vi "Actor Core.vi"(8 "error in":errorcluster, 11 "[V] User List in":refnum<class "[V] User List.lvclass">) -> (0 "error out":errorcluster, 3 "Actor out":refnum<class "Actor.lvclass">)   [LabVIEW 2020, in "[V] User List.lvlib" / "[V] User List.lvclass"]
doc: "(<B>Filename</B>: Actor Framework.lvlib:Actor.lvclass:Actor Core.vi)\n\nReceives messages to the actor, reacts to them, and initiates any error handling that may shut the actor down.\n\nDescendant classes may override this VI to append parallel tasks for the actor to complete while it handles messages. Overrides use the Call Parent Class Method node."
uses:
  [V] User List.lvclass
  C:/Program Files (x86)/National Instruments/LabVIEW 2020/vi.lib/ActorFramework/Actor/Actor.lvclass
  <vilib>/ActorFramework/Actor/Actor.lvclass
  Control/New User.ctl
  Control/Delete User.ctl
  <vilib>/ActorFramework/Actor/Actor.lvclass/Actor.ctl
  <vilib>/ActorFramework/Message Enqueuer/Message Enqueuer.lvclass/Message Enqueuer.ctl
  [V] User List.lvclass/[V] User List.ctl
  <vilib>/ActorFramework/Message Enqueuer/Init from Existing Queue.vi
  <vilib>/ActorFramework/Message Enqueuer/Enqueue.vi
  <vilib>/ActorFramework/Stop Msg/Stop Msg.lvclass
  C:/Program Files (x86)/National Instruments/LabVIEW 2020/vi.lib/ActorFramework/Message/Message.lvclass
  <vilib>/ActorFramework/Message Priority Queue/Priority Enqueue.vi
  <vilib>/ActorFramework/Message Enqueuer/Message Enqueuer.lvclass
panel:
  in  "user search":string
  in  "delete user":T1
  in  "new user":T2
  in  "user list":i32(listbox)
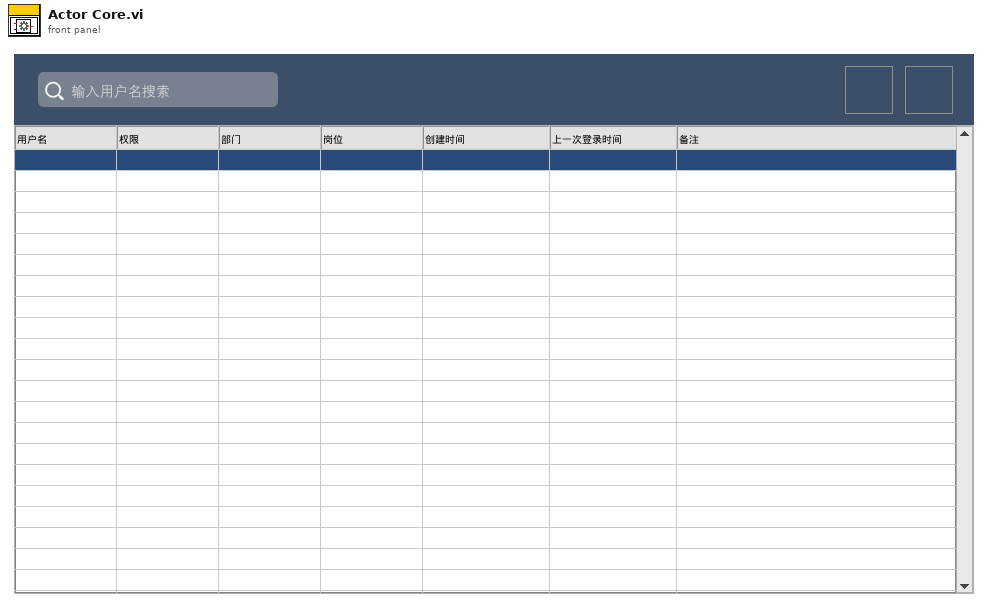
[diagram p1: front panel]
types:
  T1 = typedef "[V] User List.lvlib/[V] User List.lvclass/Delete User.ctl" = bool
  T2 = typedef "[V] User List.lvlib/[V] User List.lvclass/New User.ctl" = bool
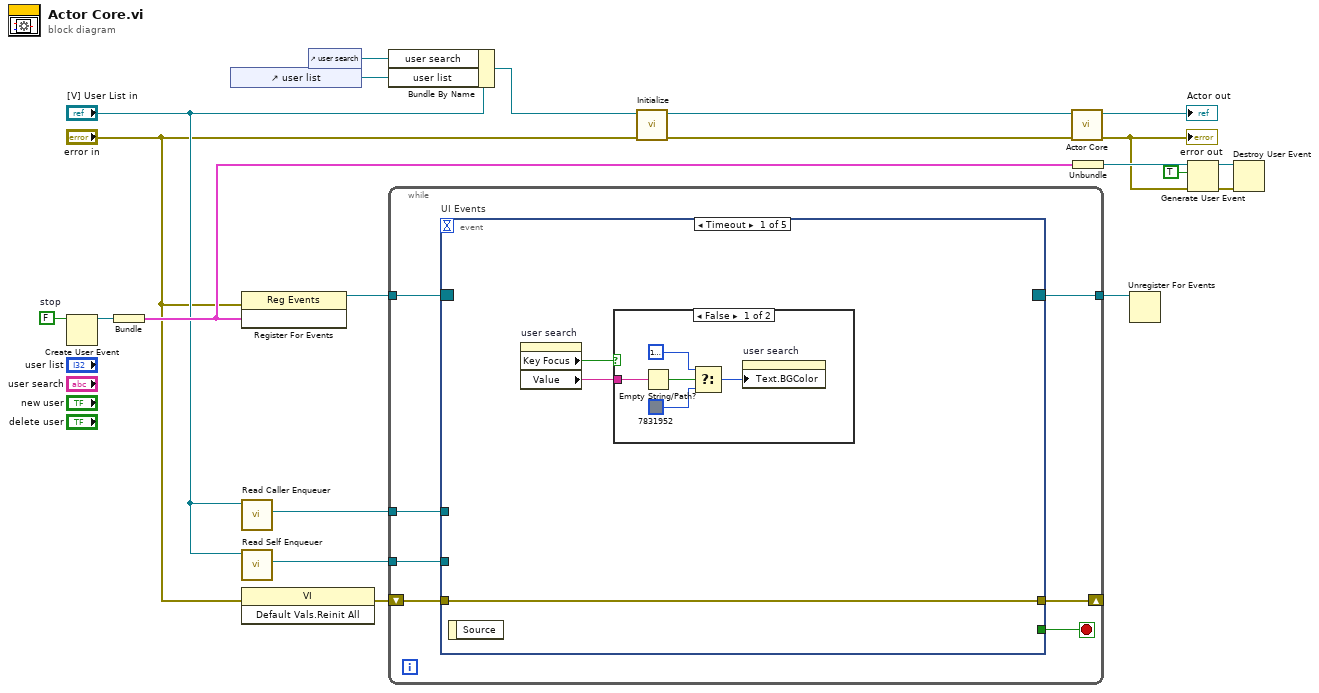
[diagram p0: block diagram]
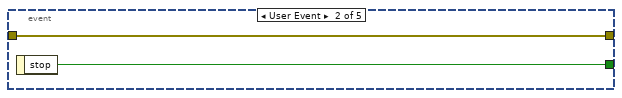
[diagram p3: hidden frame]
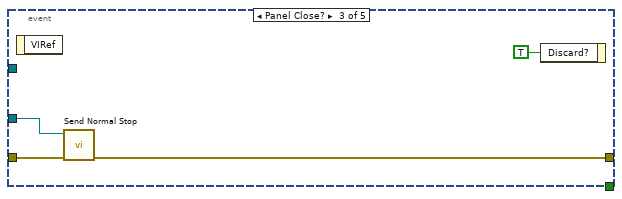
[diagram p4: hidden frame]
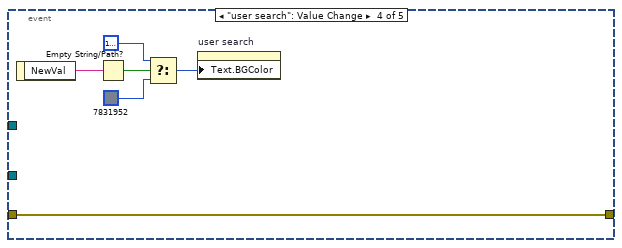
[diagram p5: hidden frame]
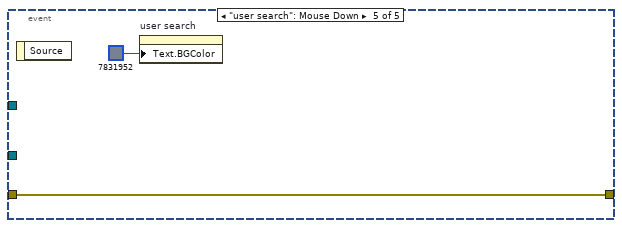
[diagram p6: hidden frame]
diagram:
  w14 = FALSE  # stop
  n1 = Create User Event(user event datatype=w14) -> (user event=w17:refnum<user-event>)  [unwired: 1 in, 1 out]
  n2 = Bundle("stop"=w17) -> (w18:cluster{"stop":refnum<user-event>})  [unwired: 1 in]
  n3 = control-ref of="user list"() -> (w6:refnum<vi>)
  n4 = register-events ("Main Register for Events")(error in="error in", w18) -> (reference out=w9:refnum<event-registration>)  [unwired: 1 in, 1 out]
  n5 = call <vilib>:"Read Caller Enqueuer.vi"("Actor"="[V] User List in") -> ("Caller Enqueuer"=w12:refnum<class "Message Enqueuer.lvclass">)  [unwired: 10 in]
  n6 = call <vilib>:"Read Self Enqueuer.vi"("Actor"="[V] User List in") -> ("Self Enqueuer"=w11:refnum<class "Message Enqueuer.lvclass">)  [unwired: 10 in]
  n7 = invoke class="VI" method="Default Vals.Reinit All"(error in="error in") -> (error out=w13:errorcluster)  [unwired: 2 in, 2 out]
  n8 = control-ref of="user search"() -> (w5:refnum<vi>)
  n9 = Bundle By Name(cluster="[V] User List in", "user search"=w5, "user list"=w6) -> (w1:refnum<class "[V] User List.lvclass">)
  n10 = while {
    tunnel: w9 -> [w28]
    tunnel: [w26] -> w10
    tunnel: w11 -> [w25]
    tunnel: w12 -> [w22]
    shift-right: [w23] -> _
    shift-left: w13 -> [w24]
    stop <- w27 stop-if-true
    n11 = event "UI Events" shown="[0] Timeout" {
      selector: w28 -> [_ _ _ _ _]
      dyn-events: [_ _ _ _ _] -> w26
      timeout: _ -> [_ _ _ _ _]
      tunnel: [_ w37 _ _ _] -> w27
      tunnel: w25 -> [_ _ w41 _ _]
      tunnel: w24 -> [w31 w38 w40 w43 w50]
      tunnel: [w31 w38 w39 w43 w50] -> w23
      tunnel: w22 -> [_ _ _ _ _]
      event Timeout {
        n12 = event-data() -> ()  [unwired: 1 in, 1 out]
        n13 = property on="user search" class="Str"() -> ("Key Focus"=w30:bool, "Value"=w29:string)  [unwired: 2 in, 2 out]
        n14 = case shown="False" w30 {
          tunnel: w29 -> [w32 _]
          frame False {
            n15 = Empty String/Path?(string/path=w32) -> (empty?=w36:bool)
            n16 = Select(t=u32 16777216 ("Text.Text Colors:Text Color"), s=w36, f=u32 7831952) -> (s? t:f=w35:u32)
            n17 = property on="user search" class="Str"("Text.BGColor"=w35) -> ()  [unwired: 2 in, 2 out]
          }
          frame True {
          }
        }
      }
      event User Event {
        n18 = event-data() -> ("stop"=w37:bool)  [unwired: 1 in]
      }
      event Panel Close? {
        n19 = event-data() -> ()  [unwired: 1 in, 1 out]
        n20 = call <vilib>:"Send Normal Stop.vi"("error in (no error)"=w40, "Message Enqueuer"=w41) -> ("error out"=w39:errorcluster)  [unwired: 9 in]
        n21 = event-data("Discard?"=TRUE) -> ()  [unwired: 1 in, 1 out]
      }
      event "user search": Value Change {
        n22 = event-data() -> ("NewVal"=w46:string)  [unwired: 1 in]
        n23 = Empty String/Path?(string/path=w46) -> (empty?=w48:bool)
        n24 = Select(t=u32 16777216 ("Text.Text Colors:Text Color"), s=w48, f=u32 7831952) -> (s? t:f=w45:u32)
        n25 = property on="user search" class="Str"("Text.BGColor"=w45) -> ()  [unwired: 2 in, 2 out]
      }
      event "user search": Mouse Down {
        n26 = event-data() -> ()  [unwired: 1 in, 1 out]
        n27 = property on="user search" class="Str"("Text.BGColor"=u32 7831952) -> ()  [unwired: 2 in, 2 out]
      }
    }
  }
  n28 = call "Initialize.vi"("error in (no error)"="error in", "[V] User List in"=w1) -> ("error out"=w4:errorcluster, "[V] User List out"=w3:refnum<class "[V] User List.lvclass">)  [unwired: 8 in]
  n29 = call-parent "Actor Core.vi"("error in"=w4, "Actor in"=w3) -> ("error out"=w8:errorcluster, "Actor out"=→"Actor out":refnum<class "Actor.lvclass">)  [unwired: 8 in]
  "error out" <- w8
  n30 = Unbundle(w18) -> ("stop"=w19:refnum<user-event>)
  n31 = Unregister For Events(event registration refnum=w10) -> ()  [unwired: 1 in, 1 out]
  n32 = Generate User Event(user event=w19, event data cluster=TRUE ("event data"), error in=w8) -> (user event out=w16:refnum<user-event>, error out=w20:errorcluster)  [unwired: 1 in]
  n33 = Destroy User Event(user event=w16, error in=w20) -> ()  [unwired: 1 out]
